vi "Main.vi"() -> ()   [LabVIEW 2018]
doc: "The myRIO Project template acquires acceleration data from the onboard accelerometer and displays the changes of acceleration values in a waveform chart."
uses:
  <vilib>/Analysis/Matrix/Datatypes/RealMatrix.ctl
  <vilib>/myRIO/Common/Instrument Driver Framework/myRIO v1.0/PWM/vis/myRIO v1.1 Open PWM.vi
  <vilib>/myRIO/Common/Instrument Driver Framework/myRIO v1.0/UART/vis/myRIO v1.0 Close UART.vi
  <vilib>/myRIO/Common/Instrument Driver Framework/Utilities/vis/Validate Channels.vi
  <vilib>/myRIO/Common/Instrument Driver Framework/myRIO v1.0/PWM/vis/myRIO v1.0 Reserve PWM.vi
  <vilib>/myRIO/Common/Instrument Driver Framework/myRIO v1.0/PWM/vis/myRIO v1.0 Build MUX Configuration PWM.vi
  <vilib>/myRIO/Common/Instrument Driver Framework/myRIO v1.0/Resource Manager/vis/myRIO v1.0 Reserve Channel List.vi
  <vilib>/myRIO/Common/Instrument Driver Framework/myRIO v1.0/Resource Manager/vis/myRIO v1.0 Create Configuration List.vi
  <vilib>/myRIO/Common/Instrument Driver Framework/myRIO v1.0/Resource Manager/vis/myRIO v1.0 Reserve Channel.vi
  <vilib>/myRIO/Common/Instrument Driver Framework/myRIO v1.0/Resource Manager/vis/myRIO v1.0 Unreserve Channel.vi
  <vilib>/myRIO/Common/Instrument Driver Framework/myRIO v1.0/Resource Manager/vis/myRIO v1.0 Build Mutex Name.vi
  <vilib>/Utility/VariantDataType/GetNumericInfo.vi
  <vilib>/Utility/error.llb/Error Cluster From Error Code.vi
  <vilib>/myRIO/Common/Instrument Driver Framework/myRIO v1.0/myRIO v1.1 Open.vi
  <vilib>/myRIO/Common/Instrument Driver Framework/Utilities/vis/IO Manager.vi
  <vilib>/myRIO/Common/Instrument Driver Framework/Utilities/vis/Configuration Manager.vi
  <vilib>/myRIO/Common/Instrument Driver Framework/myRIO v1.0/Resource Manager/vis/myRIO v1.0 Configure IO.vi
  <vilib>/myRIO/Common/Instrument Driver Framework/myRIO v1.0/myRIO v1.0 Close.vi
  <vilib>/myRIO/Common/Instrument Driver Framework/myRIO v1.0/PWM/vis/myRIO v1.0 Write PWM.vi
  <vilib>/myRIO/Common/Instrument Driver Framework/Utilities/vis/FPGA Ref Manager.vi
  <vilib>/myRIO/Common/Instrument Driver Framework/myRIO v1.0/myRIO v1.0 Reset FPGA.vi
  <vilib>/myRIO/Common/Instrument Driver Framework/myRIO v1.0/IRQ/vis/myRIO v1.0 IRQ Info FGV.vi
  <vilib>/myRIO/Common/Instrument Driver Framework/myRIO v1.0/IRQ/vis/myRIO v1.0 Timer IRQ Info FGV.vi
  <vilib>/myRIO/Common/Instrument Driver Framework/myRIO v1.0/IRQ/vis/myRIO v1.0 ISR Agent.vi
  <vilib>/myRIO/Instrument Drivers/Utilities/Utilities.lvlib
  <vilib>/myRIO/Instrument Drivers/Onboard IO/PWM/PWM.lvlib
  <vilib>/Analysis/Matrix/NI_Matrix.lvlib
panel:
  out "arm picture":refnum<vi>(3d-picture)
  out "A x B 3":T1=[[1.0, 0.0, 0.0, 0.0], [0.0, 6.123233995736766e-17, 1.0, 0.0], [0.0, -1.0, 6.123233995736766e-17, 0.0], [0.0, 0.0, 0.0, 1.0]] format="%#_2g"
  out "drawing":refnum<vi>(3d-picture)
  in  "PWM channel":tag="B/PWM0"
  in  "PWM channel 2":tag="B/PWM0"
  in  "[ESC]":bool
  in  "freq [Hz]":dbl=50.0
  out "pulse width [ms]":dbl=1.5
  out "duty cycle [%]":dbl
  in  "null offset":bool
  out "offset [%FS]":dbl
  in  "[ESC] 2":bool
  in  "freq [Hz] 2":dbl=50.0
  out "pulse width [ms] 2":dbl=1.5
  out "duty cycle [%] 2":dbl
  in  "null offset 2":bool
  out "offset [%FS] 2":dbl
  out "x arrya":dbl[][](array[numeric])
  out "phi array":dbl[][](array[numeric])
  out "third array":dbl[][](array[numeric])
  out "second array":dbl[][](array[numeric])
  out "first":dbl[][](array[numeric])
  in  "Enter initials":string
  # "Overview: The myRIO Project template acquires acceleration data from the onboard accelerometer and displays the changes of acceleration values in a waveform chart.\nInstructions:\n1. Check the myRIO target IP address in the project and make sure the target IP address is correct. \n2. Run this VI."
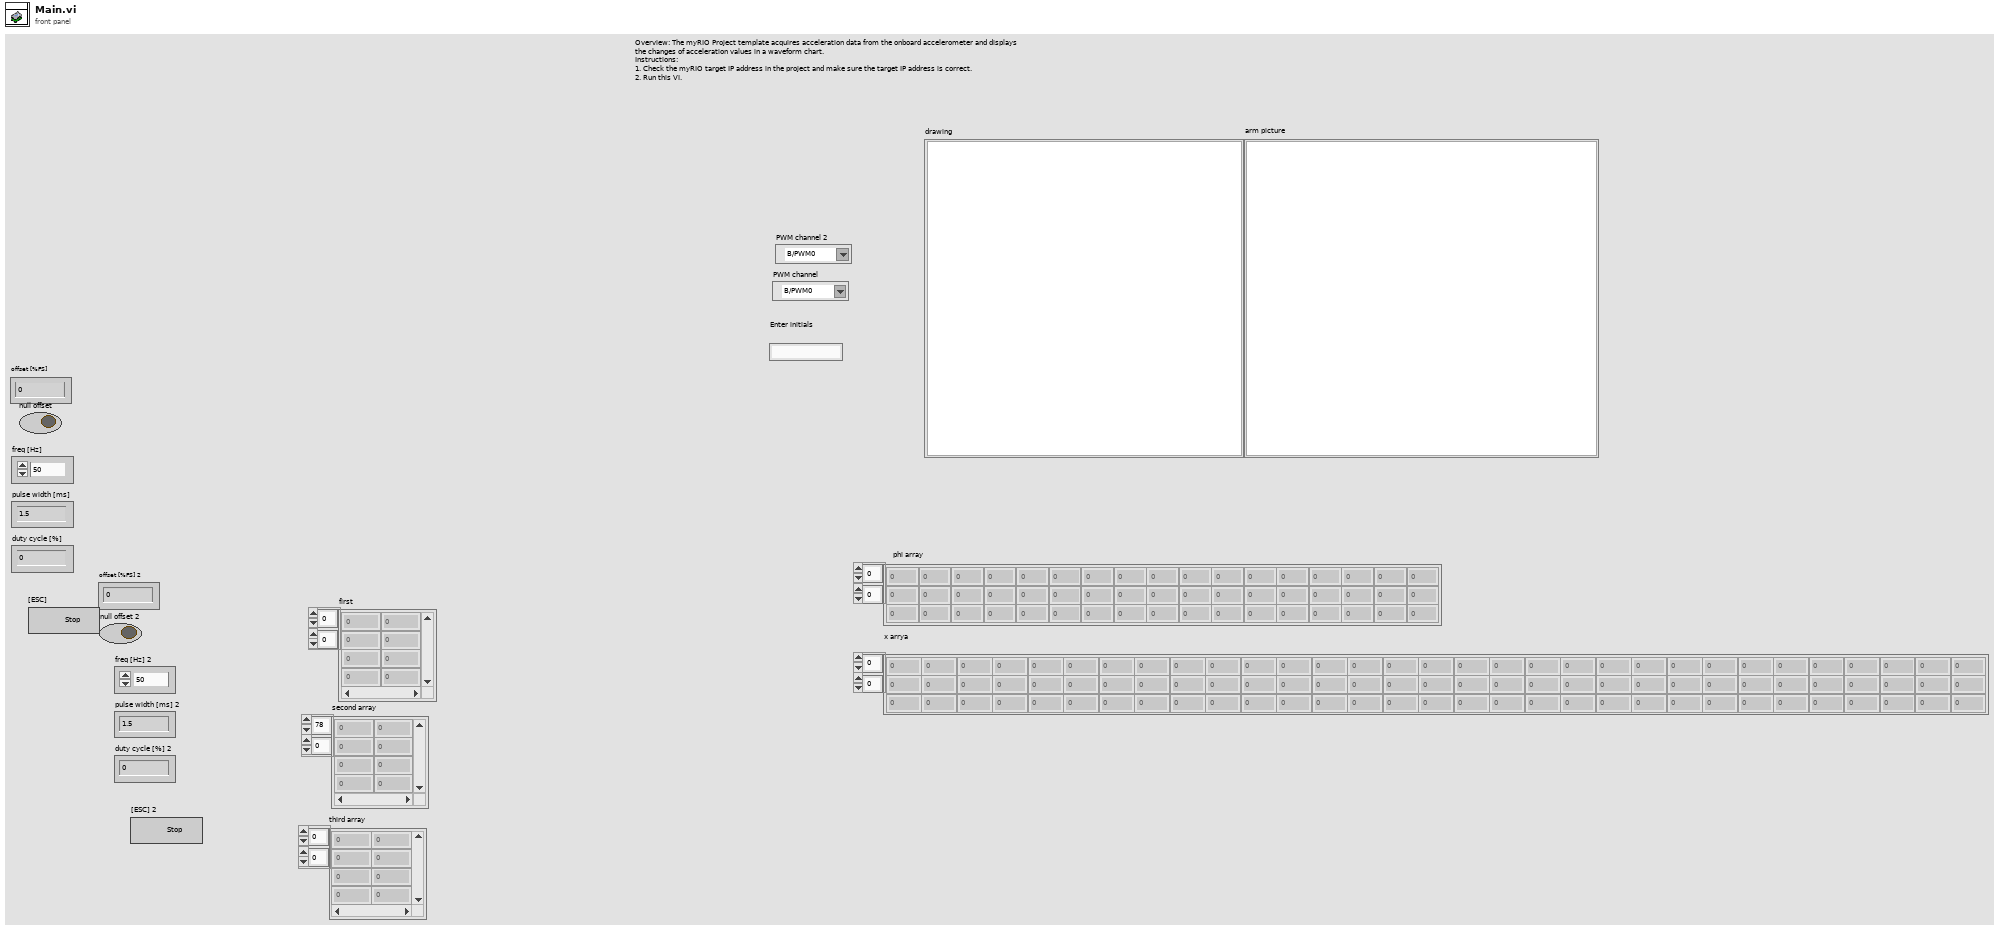
[diagram p1: front panel]
types:
  T1 = typedef "NI_Matrix.lvlib/RealMatrix.ctl" = dbl[][]
  T2 = typedef "PWM.lvlib/PWM Reference.ctl" = cluster{"myRIO Reference":T3, "PWM Channels Enum":T7, "PWM Configuration":T8}
  T3 = typedef "myRIO Generic Hardware Reference.ctl" = cluster{"myRIO Model":T4, "myRIO Hardware Reference":T5}
  T4 = typedef "Hardware Version Enum.ctl" = enum16{"Unknown", "myRIO-1900", "myRIO-1950", "roboRIO", "NI ELVIS RIO CM", "ELVIS III"}
  T5 = typedef "myRIO v1.0 Reference.ctl" = cluster{"Generic FPGA Reference":T6, "Allow multiple opens":bool}
  T6 = typedef "Generic FPGA Reference.ctl" = refnum<k20>
  T7 = typedef "PWM Channels Enum.ctl" = enum16{"Not Connected", "C/PWM0", "C/PWM1", "A/PWM0", "A/PWM1", "A/PWM2", "A/PWM3", "A/PWM4", "A/PWM5", "A/PWM6", "A/PWM7", "A/PWM8", "A/PWM9", "A/PWM10", "A/PWM11", "A/PWM12", "A/PWM13", "A/PWM14", "A/PWM15", "A/PWM16", "A/PWM17", "A/PWM18", "A/PWM19", "B/PWM0", "B/PWM1", "B/PWM2", "B/PWM3", "B/PWM4", "B/PWM5", "B/PWM6", "B/PWM7", "B/PWM8", "B/PWM9", "B/PWM10", "B/PWM11", "B/PWM12", "B/PWM13", "B/PWM14", "B/PWM15", "B/PWM16", "B/PWM17", "B/PWM18", "B/PWM19", "PWM/PWM0", "PWM/PWM1", "PWM/PWM2", "PWM/PWM3", "PWM/PWM4", "PWM/PWM5", "PWM/PWM6", "PWM/PWM7", "PWM/PWM8", "PWM/PWM9"}
  T8 = typedef "PWM.lvlib/PWM Configuration.ctl" = cluster{"Frequency":dbl, "Duty Cycle":dbl}
  T9 = cluster{"Theta":dbl, "d":dbl, "a":dbl, "alpha (degrees)":dbl}[]
  T10 = cluster{"Theta":dbl, "d":dbl, "a":dbl, "alpha (degrees)":dbl}
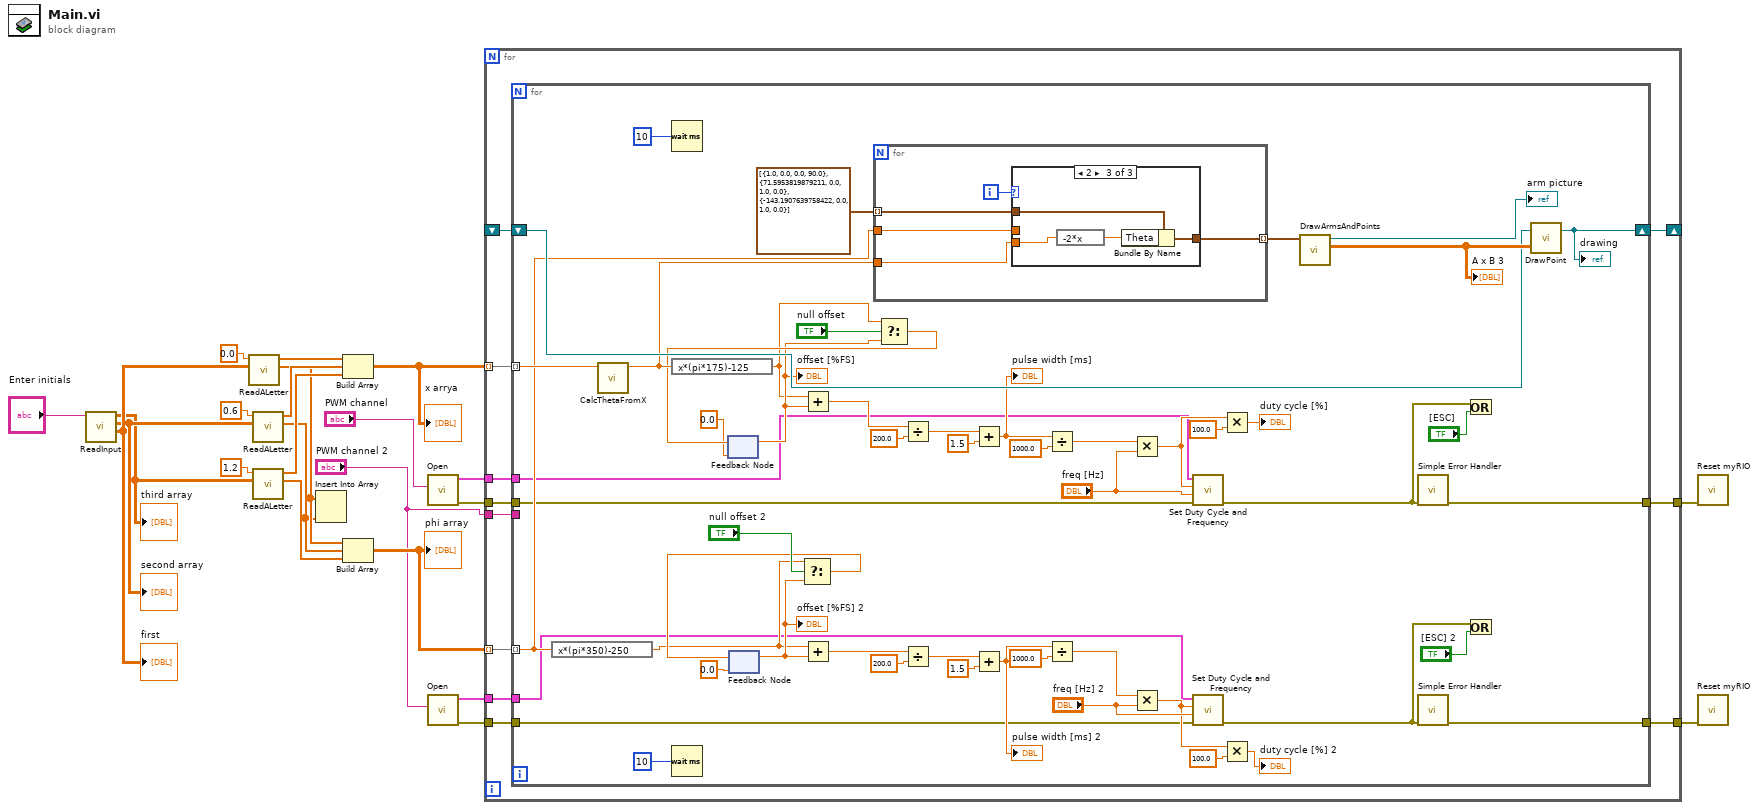
[diagram p0: block diagram]
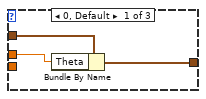
[diagram p2: hidden frame]
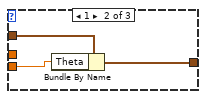
[diagram p3: hidden frame]
diagram:
  n1 = call "ReadInput.vi"("Enter initials"="Enter initials") -> ("all rows 3"=w21:dbl[][], "all rows 2"=w19:dbl[][], "all rows"=w17:dbl[][])  [unwired: 8 in]
  "first" <- w21
  "second array" <- w19
  "third array" <- w17
  n2 = call "ReadALetter.vi"("all rows 3"=w21, "x"=0.0) -> ("Array 3"=w11:dbl[], "Array 4"=w16:dbl[])  [unwired: 8 in]
  n3 = call "ReadALetter.vi"("all rows 3"=w19, "x"=0.6) -> ("Array 3"=w10:dbl[], "Array 4"=w15:dbl[])  [unwired: 8 in]
  n4 = call "ReadALetter.vi"("all rows 3"=w17, "x"=1.2) -> ("Array 3"=w9:dbl[], "Array 4"=w14:dbl[])  [unwired: 8 in]
  n5 = Insert Into Array(array=w11, new element=w10) -> ()  [unwired: 1 in, 1 out]
  n6 = Build Array(w16, w15, w14) -> (w12:dbl[][])
  "x arrya" <- w12
  n7 = Build Array(w11, w10, w9) -> (w13:dbl[][])
  "phi array" <- w13
  n8 = call <vilib>:"Open.vi"("Channel Name"="PWM channel") -> ("error out"=w8:errorcluster, "PWM Ref Out"=w7:T2)  [unwired: 9 in]
  n9 = call <vilib>:"Open.vi"("Channel Name"="PWM channel 2") -> ("error out"=w3:errorcluster, "PWM Ref Out"=w2:T2)  [unwired: 9 in]
  n10 = for {
    tunnel: w13 -> [w33] mode=indexing
    shift-right: [w34] -> _
    shift-left: _ -> [w31]
    tunnel: w12 -> [w32] mode=indexing
    tunnel: w8 -> [w30]
    tunnel: w7 -> [w29]
    tunnel: [w28] -> w5
    tunnel: [w27] -> w4
    tunnel: "PWM channel 2" -> [w26]
    tunnel: w3 -> [w25]
    tunnel: w2 -> [w24]
    n11 = for {
      tunnel: w33 -> [w79] mode=indexing
      tunnel: w32 -> [w82] mode=indexing
      shift-right: [w84] -> w34
      shift-left: w31 -> [w81]
      tunnel: w30 -> [w40]
      tunnel: w29 -> [w39]
      tunnel: [w38] -> w28
      tunnel: [w37] -> w27
      tunnel: w26 -> [_]
      tunnel: w25 -> [w36]
      tunnel: w24 -> [w35]
      n12 = expression code="x*(pi*350)-250"(w79) -> (w42:dbl)
      n13 = call "CalcThetaFromX.vi"("X"=w82) -> ("Numeric"=w80:dbl)  [unwired: 10 in]
      n14 = Wait (ms)(milliseconds to wait=u32 10) -> ()  [unwired: 1 out]
      n15 = expression code="x*(pi*175)-125"(w80) -> (w61:dbl)
      n16 = Wait (ms)(milliseconds to wait=u32 10) -> ()  [unwired: 1 out]
      n17 = feedback #1(0.0 ("position [%FS]")) -> (w67:dbl)
      "offset [%FS]" <- w67
      n18 = feedback #2(0.0 ("position [%FS]")) -> (w48:dbl)
      "offset [%FS] 2" <- w48
      n19 = Select(t=w42, s="null offset 2", f=w48) -> (s? t:f=w50:dbl)
      n20 = feedback-in #2(w50) -> ()
      n21 = Add(x=w61, y=w67) -> (x+y=w68:dbl)
      n22 = Add(x=w42, y=w48) -> (x+y=w49:dbl)
      n23 = for {
        tunnel: T9 [{"Theta"=1.0, "d"=0.0, "a"=0.0, "alpha (degrees)"=90.0}, {"Theta"=71.5953819879211, "d"=0.0, "a"=1.0, "alpha (degrees)"=0.0}, {"Theta"=-143.1907639758422, "d"=0.0, "a"=1.0, "alpha (degrees)"=0.0}] ("Joints") -> [w92] mode=indexing
        tunnel: [w91] -> w86 mode=indexing
        tunnel: w80 -> [w89]
        tunnel: w79 -> [w88]
        i -> [w90]
        n24 = case shown="2" w90 {
          tunnel: w89 -> [_ w97 w101]
          tunnel: w92 -> [w95 w98 w102]
          tunnel: [w93 w96 w100] -> w91
          tunnel: w88 -> [w94 _ _]
          frame 0, Default {
            n25 = Bundle By Name(cluster=w95, "Theta"=w94) -> (w93:T10)
          }
          frame 1 {
            n26 = Bundle By Name(cluster=w98, "Theta"=w97) -> (w96:T10)
          }
          frame 2 {
            n27 = expression code="-2*x"(w101) -> (w99:dbl)
            n28 = Bundle By Name(cluster=w102, "Theta"=w99) -> (w100:T10)
          }
        }
      }
      n29 = Select(t=w61, s="null offset", f=w67) -> (s? t:f=w69:dbl)
      n30 = feedback-in #1(w69) -> ()
      n31 = Divide(x=w68, y=200.0) -> (x/y=w75:dbl)
      n32 = Divide(x=w49, y=200.0) -> (x/y=w56:dbl)
      n33 = Add(x=w75, y=1.5) -> (x+y=w73:dbl)
      "pulse width [ms]" <- w73
      n34 = Add(x=w56, y=1.5) -> (x+y=w54:dbl)
      "pulse width [ms] 2" <- w54
      n35 = Divide(x=w73, y=1000.0) -> (x/y=w66:dbl)
      n36 = Divide(x=w54, y=1000.0) -> (x/y=w47:dbl)
      n37 = Multiply(x=w66, y="freq [Hz]") -> (x*y=w63:dbl)
      n38 = Multiply(x=w47, y="freq [Hz] 2") -> (x*y=w44:dbl)
      n39 = call <vilib>:"Set Duty Cycle and Frequency.vi"("error in (no error)"=w40, "Frequency [Hz]"="freq [Hz]", "Duty Cycle"=w63, "PWM Ref In"=w39) -> ("error out"=w60:errorcluster)  [unwired: 5 in, 1 out]
      n40 = call <vilib>:"Set Duty Cycle and Frequency.vi"("error in (no error)"=w36, "Frequency [Hz]"="freq [Hz] 2", "Duty Cycle"=w44, "PWM Ref In"=w35) -> ("error out"=w41:errorcluster)  [unwired: 5 in, 1 out]
      n41 = Multiply(x=w63, y=100.0) -> (x*y=→"duty cycle [%]":dbl)
      n42 = Multiply(x=w44, y=100.0) -> (x*y=→"duty cycle [%] 2":dbl)
      n43 = call "DrawArmsAndPoints.vi"("Array"=w86) -> ("A x B"=w85:T1, "SceneObject out"=→"arm picture":refnum<vi>)  [unwired: 9 in]
      "A x B 3" <- w85
      n44 = call <vilib>:"Simple Error Handler.vi"("error in (no error)"=w60) -> ("error out"=w38:errorcluster)  [unwired: 4 in, 4 out]
      n45 = call <vilib>:"Simple Error Handler.vi"("error in (no error)"=w41) -> ("error out"=w37:errorcluster)  [unwired: 4 in, 4 out]
      n46 = Or(x=w60, y="[ESC]") -> ()  [unwired: 1 out]
      n47 = Or(x=w41, y="[ESC] 2") -> ()  [unwired: 1 out]
      n48 = call "DrawPoint.vi"("Start"=w85, "Stage in"=w81) -> ("Stage out"=w84:refnum<vi>)  [unwired: 1 in]
      "drawing" <- w84
    }
  }
  n49 = call <vilib>:"Reset myRIO.vi"("error in (no error)"=w5) -> ()  [unwired: 10 in, 1 out]
  n50 = call <vilib>:"Reset myRIO.vi"("error in (no error)"=w4) -> ()  [unwired: 10 in, 1 out]
